vi "lockLEDPWM.vi"(8 "error in (no error)":errorcluster, 10 "PD Targets":dbl[](array[numeric]), 11 "Arduino session":refnum<visa-resource-name>) -> (0 "error out":errorcluster, 1 "LED vector":bool[](array[boolean]), 2 "Locked Vector":bool[](array[boolean]), 3 "Arduino session":refnum<visa-resource-name>)   [LabVIEW 2017]
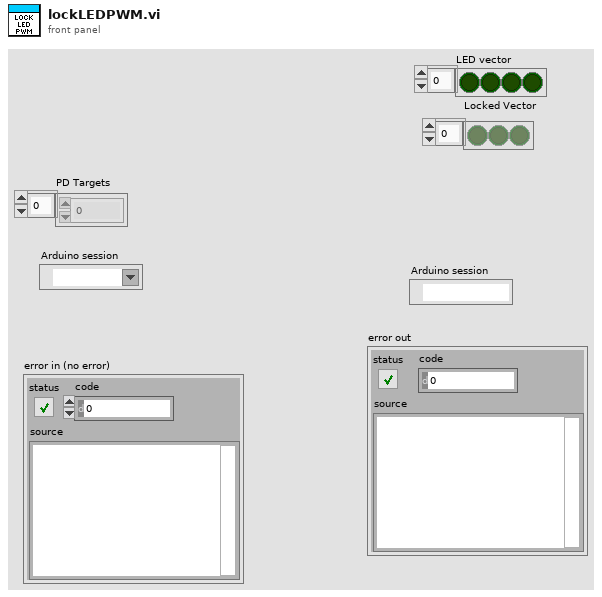
[diagram p1: front panel]
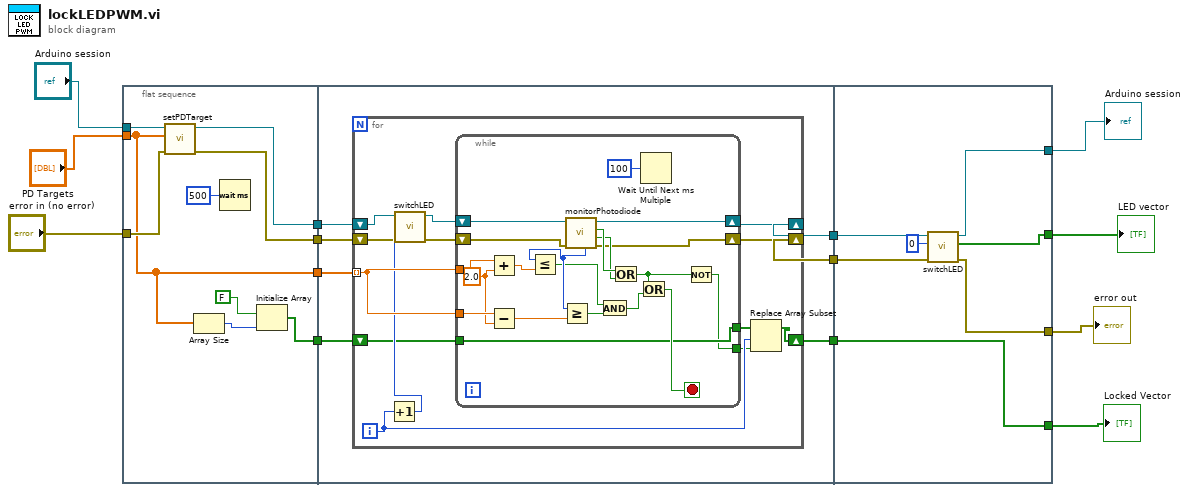
[diagram p0: block diagram]
diagram:
  n1 = flat-sequence {
    tunnel: "Arduino session" -> [w23]
    tunnel: "PD Targets" -> [w18]
    tunnel: "error in (no error)" -> [w22]
    tunnel: [w20] -> w11
    tunnel: [w18] -> w10
    tunnel: [w19] -> w9
    tunnel: [w15] -> w3
    tunnel: w11 -> [w30]
    tunnel: w10 -> [w29]
    tunnel: w9 -> [w28]
    tunnel: [w27] -> w8
    tunnel: [w26] -> w7
    tunnel: w3 -> [w25]
    tunnel: [w24] -> w1
    tunnel: w8 -> [w70]
    tunnel: w7 -> [w69]
    tunnel: [w67] -> w6
    tunnel: [w66] -> w5
    tunnel: [w65] -> w4
    tunnel: [w64] -> w2
    tunnel: w1 -> [w64]
    frame #0 {
      n2 = call "setPDTarget.vi"("error in (no error)"=w22, "Photodiode Targets"=w18, "Arduino session"=w23) -> ("error out"=w19:errorcluster, "Arduino session"=w20:refnum<visa-resource-name>)  [unwired: 7 in]
      n3 = Array Size(array=w18) -> (size(s)=w17:i32)
      n4 = Wait (ms)(milliseconds to wait=u32 500) -> ()  [unwired: 1 out]
      n5 = Initialize Array(FALSE, w17) -> (w15:bool[])
    }
    frame #1 {
      n6 = for {
        shift-right: [w43] -> w27
        shift-left: w30 -> [w40]
        tunnel: w29 -> [w42] mode=indexing
        shift-right: [w36] -> w26
        shift-left: w28 -> [w38]
        shift-right: [w31] -> w24
        shift-left: w25 -> [w34]
        i -> [w33]
        n7 = Increment(x=w33) -> (x+1=w41:i32)
        n8 = call "switchLED.vi"("error in (no error)"=w38, "Which LED"=w41, "Arduino session"=w40) -> ("error out"=w37:errorcluster, "Arduino session"=w39:refnum<visa-resource-name>)  [unwired: 6 in, 1 out]
        n9 = while {
          shift-right: [w61] -> w43
          shift-left: w39 -> [w62]
          tunnel: w42 -> [w58]
          tunnel: w42 -> [w56]
          shift-right: [w47] -> w36
          shift-left: w37 -> [w48]
          tunnel: [w45] -> w35
          tunnel: w34 -> [w45]
          tunnel: [w44] -> w32
          stop <- w49 stop-if-true
          w55 = 2.0 ("y")
          n10 = Add(x=w58, y=w55) -> (x+y=w54:dbl)
          n11 = Subtract(x=w56, y=w55) -> (x-y=w57:dbl)
          n12 = call "monitorPhotodiode.vi"("error in (no error)"=w48, "Arduino session"=w62) -> ("error out"=w47:errorcluster, "Photodiode Warning"=w59:bool, "LED Warning"=w60:bool, "Arduino session"=w61:refnum<visa-resource-name>, "PD Value"=w53:i32)  [unwired: 5 in]
          n13 = Less Or Equal?(x=w53, y=w54) -> (x <= y?=w51:bool)
          n14 = Greater Or Equal?(x=w53, y=w57) -> (x >= y?=w52:bool)
          n15 = And(x=w51, y=w52) -> (x .and. y?=w50:bool)
          n16 = Or(x=w60, y=w59) -> (x .or. y?=w46:bool)
          n17 = Or(x=w46, y=w50) -> (x .or. y?=w49:bool)
          n18 = Wait Until Next ms Multiple(millisecond multiple=u32 100) -> ()  [unwired: 1 out]
          n19 = Not(x=w46) -> (.not. x?=w44:bool)
        }
        n20 = Replace Array Subset(array=w35, new element=w32, index=w33) -> (w31:bool[])
      }
    }
    frame #2 {
      n21 = call "switchLED.vi"("error in (no error)"=w69, "Which LED"=u8 0, "Arduino session"=w70) -> ("error out"=w66:errorcluster, "LED vector"=w65:bool[], "Arduino session"=w67:refnum<visa-resource-name>)  [unwired: 6 in]
    }
  }
  "Arduino session" <- w6
  "error out" <- w5
  "LED vector" <- w4
  "Locked Vector" <- w2
